vi "Set Home Impl.vi"(8 "error in (no error)":errorcluster, 11 "Ludl Stage in":refnum<class "Ludl Stage.lvclass">) -> (0 "error out":errorcluster, 3 "Ludl Stage out":refnum<class "Ludl Stage.lvclass">)   [LabVIEW 2023, in "Ludl Stage.lvlib" / "Ludl Stage.lvclass"]
uses:
  Ludl Stage.lvclass
  Ludl Stage.lvclass/Ludl Stage.ctl
  Stage Controller/Stage Controller.lvlib
  Resources/GLOBAL/GLOBAL Debug.vi
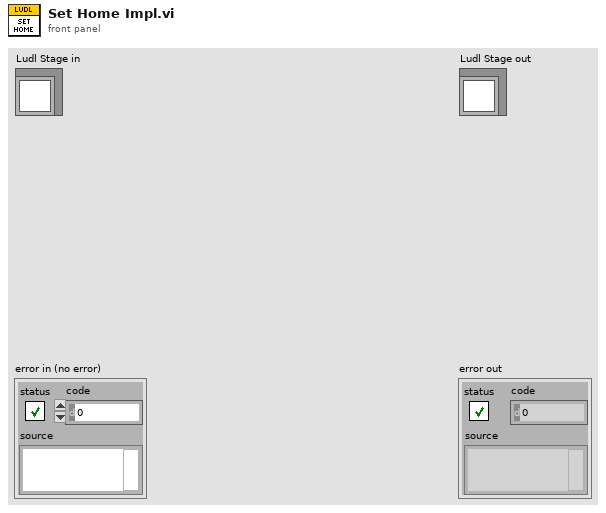
[diagram p1: front panel]
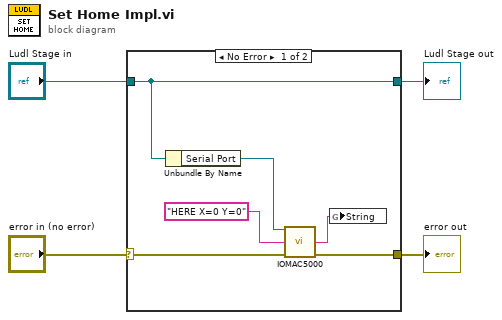
[diagram p0: block diagram]
diagram:
  n1 = case shown="No Error" "error in (no error)" {
    selector: "error in (no error)" -> [w7 w12]
    tunnel: [w8 w12] -> w4
    tunnel: "Ludl Stage in" -> [w5 w11]
    tunnel: [w5 w11] -> w1
    frame No Error {
      n2 = Unbundle By Name(w5) -> ("Serial Port"=w6:refnum<visa-resource-name>)
      n3 = call "IOMAC5000.vi"("VISA  IN"=w6, "Command (to ctlr)"="HERE X=0 Y=0" ("true string"), "error in"=w7) -> ("Raw Response"=w9:string, "error out"=w8:errorcluster)  [unwired: 9 in, 2 out]
      n4 = global write "GLOBAL Debug.vi" "String"(w9) -> ()
    }
    frame Error {
    }
  }
  "error out" <- w4
  "Ludl Stage out" <- w1
